vi "数组表转换成电子表.vi"() -> ()   [LabVIEW 2018]
panel:
  out "字符串 2":string
  in  "组合框":string(combo)
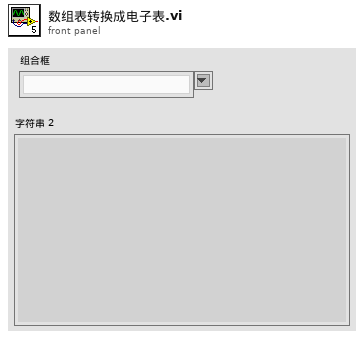
[diagram p1: front panel]
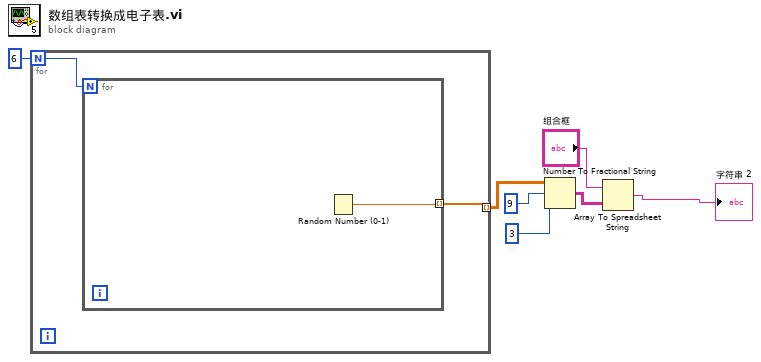
[diagram p0: block diagram]
diagram:
  n1 = for {
    N: 6 -> [w9]
    tunnel: [w8] -> w6 mode=indexing
    n2 = for {
      N: w9 -> [_]
      tunnel: [w10] -> w8 mode=indexing
      n3 = Random Number (0-1)() -> (number: 0 to 1=w10:dbl)
    }
  }
  n4 = Number To Fractional String(number=w6, width (-)=i16 9 ("宽度(-)"), precision (6)=i16 3 ("精度(6)")) -> (F-format string=w3:string[][])  [unwired: 1 in]
  n5 = Array To Spreadsheet String(array=w3, 3:"组合框") -> (spreadsheet string=→"字符串 2":string)  [unwired: 1 in]
